vi "createOutboundChannel.vi"(8 "error in (no error)":errorcluster, 10 "redirect":string, 11 "Connection.LocalQueue in":refnum<class "Connection.LocalQueue.lvclass">) -> (0 "error out":errorcluster, 3 "Connection.LocalQueue out":refnum<class "Connection.LocalQueue.lvclass">)   [LabVIEW 2013, in "Connection.Queue_GOSPL.lvlib" / "Connection.LocalQueue.lvclass"]
uses:
  Connection.LocalQueue.lvclass
  Connection/Connection.lvclass
  Connection/Connection.lvclass/Connection.ctl
  Connection.LocalQueue.lvclass/Connection.LocalQueue.ctl
panel:
  out "Numeric":i32
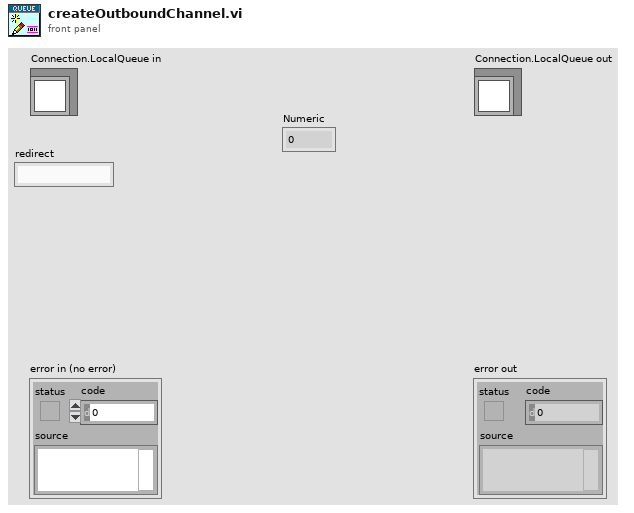
[diagram p1: front panel]
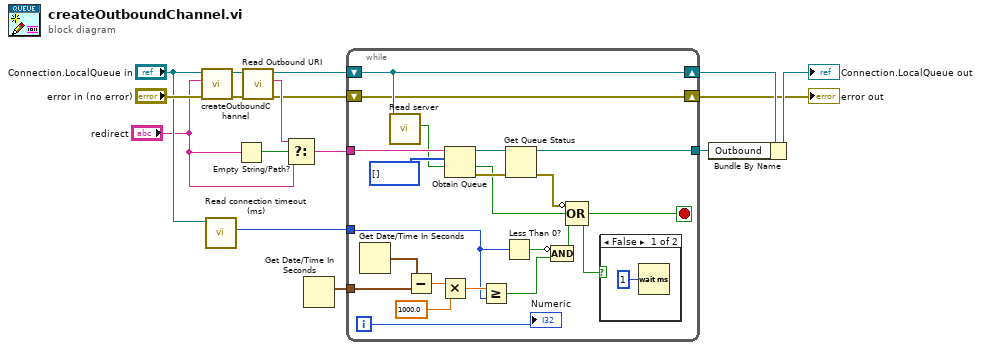
[diagram p0: block diagram]
diagram:
  n1 = call-parent "createOutboundChannel.vi"("error in (no error)"="error in (no error)", "redirect"="redirect", "Connection in"="Connection.LocalQueue in") -> ("error out"=w5:errorcluster, "Connection out"=w10:refnum<class "Connection.LocalQueue.lvclass">)  [unwired: 7 in]
  n2 = call "Read connection timeout (ms).vi"("Connection in"="Connection.LocalQueue in") -> ("connection timeout (ms)"=w6:i32)  [unwired: 8 in, 2 out]
  n3 = Empty String/Path?(string/path="redirect") -> (empty?=w13:bool)
  n4 = call "Read Outbound URI.vi"("Connection in"=w10) -> ("Outbound URI"=w12:string, "Connection out"=w8:refnum<class "Connection.LocalQueue.lvclass">)  [unwired: 9 in]
  n5 = Select(t=w12, s=w13, f="redirect") -> (s? t:f=w11:string)
  n6 = Get Date/Time In Seconds() -> (seconds since 1Jan1904=w3:timestamp)
  n7 = while {
    tunnel: w11 -> [w35]
    tunnel: [w32] -> w1
    shift-right: [w31] -> w7
    shift-left: w8 -> [w31]
    tunnel: w6 -> [w18]
    shift-right: [w30] -> w4
    shift-left: w5 -> [w30]
    tunnel: w3 -> [w26]
    i -> [w16]
    stop <- w17 stop-if-true
    n8 = Get Date/Time In Seconds() -> (seconds since 1Jan1904=w25:timestamp)
    n9 = call "Read server.vi"("Connection in"=w31) -> ("server"=w34:bool)  [unwired: 9 in, 1 out]
    n10 = Subtract(x=w25, y=w26) -> (x-y=w24:dbl)
    n11 = Multiply(x=w24, y=1000.0) -> (x*y=w22:dbl)
    n12 = Obtain Queue(name (unnamed)=w35, element data type=u8[] [] ("Bytes"), create if not found? (T)=w34) -> (queue out=w33:refnum<queue>, created new?=w27:bool, error out=w29:errorcluster)  [unwired: 2 in]
    n13 = Greater Or Equal?(x=w22, y=w18) -> (x >= y?=w21:bool)
    n14 = Less Than 0?(x=w18) -> (x < 0?=w19:bool)
    n15 = Get Queue Status(queue=w33, error in (no error)=w29) -> (queue out=w32:refnum<queue>, error out=w28:errorcluster)  [unwired: 1 in, 6 out]
    n16 = Compound Arithmetic op=AND(invert w19, w21) -> (w20:bool)
    n17 = Compound Arithmetic op=OR(invert w28, w27, w20) -> (w17:bool)
    n18 = case shown="False" w17 {
      frame False {
        n19 = Wait (ms)(milliseconds to wait=u32 1) -> ()  [unwired: 1 out]
      }
      frame True {
      }
    }
    "Numeric" <- w16
  }
  "error out" <- w4
  n20 = Bundle By Name(cluster=w7, "Outbound"=w1) -> (→"Connection.LocalQueue out":refnum<class "Connection.LocalQueue.lvclass">)
